vi "Steer Control Loop (Periodic).vi"(0 "Front Left Steer":T4={"DeviceStatus"={"status"=FALSE, "code"=0, "source"=""}, "Type"=enum."PWM", "PWM"={"Digital Module"=enum."Digital Module 1", "PWM Channel"=enum."Invalid", "DeadBand"={"Name"="", "maxPositivePwm"=0, "minPositivePwm"=0, "centerPwm"=0, "maxNegativePwm"=0, "minNegativePwm"=0, "angularRange"=0}}, "CAN"={"Device Number"=0, "Control Mode"=enum."Percent VBus", "Semaphore"=refnum, "Max Vout"=12.0}, "Invert"=FALSE, "TransformRef"=refnum, "InvTransformRef"=refnum}, 1 "Front Right Steer":T4={"DeviceStatus"={"status"=FALSE, "code"=0, "source"=""}, "Type"=enum."PWM", "PWM"={"Digital Module"=enum."Digital Module 1", "PWM Channel"=enum."Invalid", "DeadBand"={"Name"="", "maxPositivePwm"=0, "minPositivePwm"=0, "centerPwm"=0, "maxNegativePwm"=0, "minNegativePwm"=0, "angularRange"=0}}, "CAN"={"Device Number"=0, "Control Mode"=enum."Percent VBus", "Semaphore"=refnum, "Max Vout"=12.0}, "Invert"=FALSE, "TransformRef"=refnum, "InvTransformRef"=refnum}, 2 "Rear Left Steer":T4={"DeviceStatus"={"status"=FALSE, "code"=0, "source"=""}, "Type"=enum."PWM", "PWM"={"Digital Module"=enum."Digital Module 1", "PWM Channel"=enum."Invalid", "DeadBand"={"Name"="", "maxPositivePwm"=0, "minPositivePwm"=0, "centerPwm"=0, "maxNegativePwm"=0, "minNegativePwm"=0, "angularRange"=0}}, "CAN"={"Device Number"=0, "Control Mode"=enum."Percent VBus", "Semaphore"=refnum, "Max Vout"=12.0}, "Invert"=FALSE, "TransformRef"=refnum, "InvTransformRef"=refnum}, 3 "Rear Right Steer":T4={"DeviceStatus"={"status"=FALSE, "code"=0, "source"=""}, "Type"=enum."PWM", "PWM"={"Digital Module"=enum."Digital Module 1", "PWM Channel"=enum."Invalid", "DeadBand"={"Name"="", "maxPositivePwm"=0, "minPositivePwm"=0, "centerPwm"=0, "maxNegativePwm"=0, "minNegativePwm"=0, "angularRange"=0}}, "CAN"={"Device Number"=0, "Control Mode"=enum."Percent VBus", "Semaphore"=refnum, "Max Vout"=12.0}, "Invert"=FALSE, "TransformRef"=refnum, "InvTransformRef"=refnum}, 4 "Front Left Pot":T1, 5 "Front Right Pot":T1, 6 "Rear Left Pot":T1, 7 "Rear Right Pot":T1, 10 "PID gains (strong motor)":T11={"proportional gain (Kc)"=4.0, "integral time (Ti, min)"=0.0, "derivative time (Td, min)"=0.0} {"derivative time (Td, min)" format="%.6f"; "integral time (Ti, min)" format="%.3f"; "proportional gain (Kc)" format="%.3f"}, 14 "PID gains (weak motor)":T11={"proportional gain (Kc)"=8.0, "integral time (Ti, min)"=0.0, "derivative time (Td, min)"=0.0} {"derivative time (Td, min)" format="%.6f"; "integral time (Ti, min)" format="%.3f"; "proportional gain (Kc)" format="%.3f"}) -> ()   [LabVIEW 2012]
uses:
  <vilib>/Rock Robotics/WPI/MotorControl/WPI_MotorControlDeviceRef.ctl
  <vilib>/Rock Robotics/SystemInterfaces/Typedef/FPGA_TypedefDigitalModule.ctl
  <vilib>/Rock Robotics/SystemInterfaces/DIO/FPGA_DIOPWMChannel.ctl
  <vilib>/Rock Robotics/WPI/PWM/WPI_PWMDeadband.ctl
  <vilib>/Rock Robotics/WPI/CAN/Jaguar/SubVIs/WPI_CANJaguar_ControlMode.ctl
  <vilib>/Rock Robotics/WPI/PWM/WPI_PWMTransform_ConPane.ctl
  <vilib>/Rock Robotics/WPI/AnalogChannel/WPI_AnalogChannelDevRef.ctl
  <vilib>/Rock Robotics/SystemInterfaces/Typedef/FPGA_TypedefAnalogModule.ctl
  <vilib>/Rock Robotics/SystemInterfaces/AI/FPGA_AIChannel.ctl
  Controls/Sensor.ctl
  Globals/Jaguar Commands.vi
  Globals/Max Steer Voltage.vi
  Globals/Robot Turning.vi
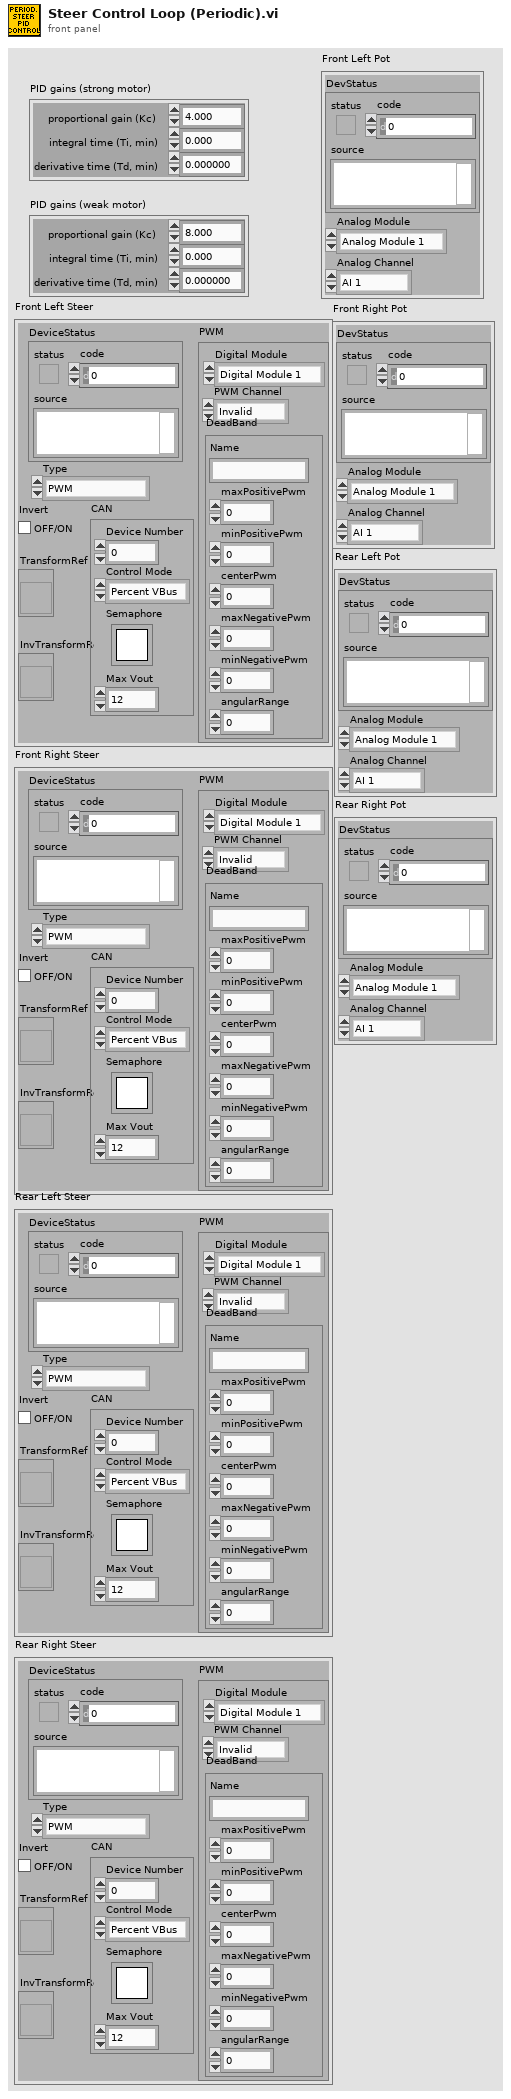
[diagram p1: front panel]
types:
  T1 = typedef "WPI_AnalogChannelDevRef.ctl" = cluster{"DevStatus":errorcluster, "Analog Module":T2, "Analog Channel":T3}
  T2 = typedef "FPGA_TypedefAnalogModule.ctl" = enum16{"Analog Module 1", "Analog Module 2"}
  T3 = typedef "FPGA_AIChannel.ctl" = enum8{"AI 1", "AI 2", "AI 3", "AI 4", "AI 5", "AI 6", "AI 7", "AI 8", "Invalid"}
  T4 = typedef "WPI_MotorControlDeviceRef.ctl" = cluster{"DeviceStatus":errorcluster, "Type":enum16{"PWM", "CAN"}, "PWM":cluster{"Digital Module":T5, "PWM Channel":T6, "DeadBand":T7}, "CAN":cluster{"Device Number":u8, "Control Mode":T8, "Semaphore":T9, "Max Vout":dbl}, "Invert":bool, "TransformRef":T10, "InvTransformRef":T10}
  T5 = typedef "FPGA_TypedefDigitalModule.ctl" = enum16{"Digital Module 1", "Digital Module 2"}
  T6 = typedef "FPGA_DIOPWMChannel.ctl" = enum8{"PWM 1", "PWM 2", "PWM 3", "PWM 4", "PWM 5", "PWM 6", "PWM 7", "PWM 8", "PWM 9", "PWM 10", "Invalid"}
  T7 = typedef "WPI_PWMDeadband.ctl" = cluster{"Name":string, "maxPositivePwm":i32, "minPositivePwm":i32, "centerPwm":i32, "maxNegativePwm":i32, "minNegativePwm":i32, "angularRange":u16}
  T8 = typedef "WPI_CANJaguar_ControlMode.ctl" = enum8{"Percent VBus", "Current", "Speed", "Position", "Voltage"}
  T9 = typedef "Semaphore RefNum" = refnum<k1>
  T10 = typedef "WPI_PWMTransform_ConPane.ctl" = refnum<vi>
  T11 = cluster{"proportional gain (Kc)":dbl, "integral time (Ti, min)":dbl, "derivative time (Td, min)":dbl}
  T12 = typedef "Sensor.ctl" = enum16{"Potentiometer", "Encoder"}
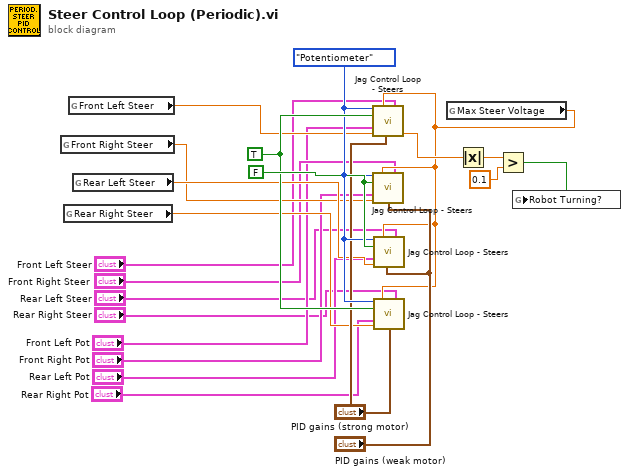
[diagram p0: block diagram]
diagram:
  w18 = FALSE ("Strong wheel?")
  w17 = TRUE
  w16 = Sensor."Potentiometer" ("Sensor")
  n1 = global read "Jaguar Commands.vi" "Front Right Steer"() -> (w10:dbl)
  n2 = global read "Jaguar Commands.vi" "Rear Right Steer"() -> (w12:dbl)
  n3 = global read "Jaguar Commands.vi" "Front Left Steer"() -> (w9:dbl)
  n4 = global read "Jaguar Commands.vi" "Rear Left Steer"() -> (w11:dbl)
  n5 = global read "Max Steer Voltage.vi" "Max Steer Voltage"() -> (w13:dbl)
  n6 = call "Jag Control Loop - Steers.vi"("Sensor"=w16, "Voltage Limit"=w13, "MotorControlDevRef"="Front Left Steer", "Strong wheel?"=w17, "AIDeviceRef"="Front Left Pot", "Command"=w9, "PID gains"="PID gains (strong motor)") -> ("Motor Output"=w19:dbl)  [unwired: 7 in, 1 out]
  n7 = call "Jag Control Loop - Steers.vi"("Sensor"=w16, "Voltage Limit"=w13, "MotorControlDevRef"="Front Right Steer", "Strong wheel?"=w18, "AIDeviceRef"="Front Right Pot", "Command"=w10, "PID gains"="PID gains (weak motor)") -> ()  [unwired: 7 in, 2 out]
  n8 = call "Jag Control Loop - Steers.vi"("Sensor"=w16, "Voltage Limit"=w13, "MotorControlDevRef"="Rear Left Steer", "Strong wheel?"=w18, "AIDeviceRef"="Rear Left Pot", "Command"=w11, "PID gains"="PID gains (weak motor)") -> ()  [unwired: 7 in, 2 out]
  n9 = call "Jag Control Loop - Steers.vi"("Sensor"=w16, "Voltage Limit"=w13, "MotorControlDevRef"="Rear Right Steer", "Strong wheel?"=w17, "AIDeviceRef"="Rear Right Pot", "Command"=w12, "PID gains"="PID gains (strong motor)") -> ()  [unwired: 7 in, 2 out]
  n10 = Absolute Value(x=w19) -> (abs(x)=w20:dbl)
  n11 = Greater?(x=w20, y=0.1) -> (0:w22:bool)
  n12 = global write "Robot Turning.vi" "Robot Turning?"(w22) -> ()
